vi "set_up_NS_queue.vi"(8 "error in (no error)":errorcluster, 10 "target":T1, 11 "StreamingBase in":refnum<class "StreamingBase.lvclass">) -> (0 "error out":errorcluster, 3 "StreamingBase out":refnum<class "StreamingBase.lvclass">)   [LabVIEW 2011, in "StreamingBase.lvclass"]
uses:
  StreamingBase.lvclass
  component_specification_cluster.ctl
  observer_cluster.ctl
  StreamingBase.lvclass/StreamingBase.ctl
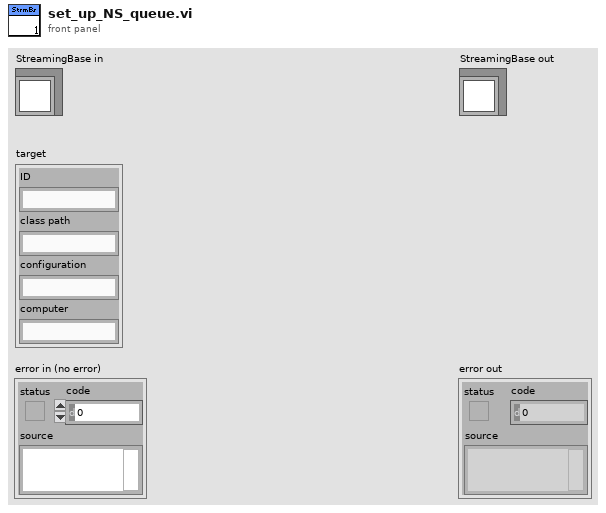
[diagram p1: front panel]
types:
  T1 = typedef "StreamingBase.lvclass/component_specification_cluster.ctl" = cluster{"ID":string, "class path":string, "configuration":string, "computer":string}
  T2 = typedef "StreamingBase.lvclass/observer_cluster.ctl" = cluster{"writer endpoint":refnum<k21>, "reader endpoint":refnum<k21>}
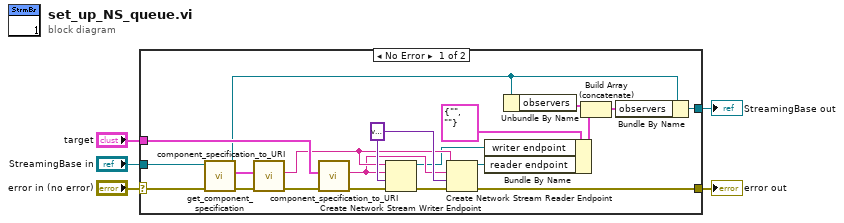
[diagram p0: block diagram]
diagram:
  n1 = case shown="No Error" "error in (no error)" {
    selector: "error in (no error)" -> [w25 w27]
    tunnel: [w22 w27] -> w4
    tunnel: [w6 w26] -> w2
    tunnel: "StreamingBase in" -> [w16 w26]
    tunnel: "target" -> [w17 _]
    frame No Error {
      w24 = variant ("variant")
      n2 = call-dynamic "get_component_specification.vi"("error in (no error)"=w25, "StreamingBase in"=w16) -> ("error out"=w21:errorcluster, "component specification"=w20:T1, "StreamingBase out"=w7:refnum<class "StreamingBase.lvclass">)  [unwired: 7 in]
      n3 = call "component_specification_to_URI.vi"("error in (no error)"=w21, "component specification"=w20) -> ("error out"=w19:errorcluster, "URI"=w15:string)  [unwired: 8 in]
      n4 = call "component_specification_to_URI.vi"("error in (no error)"=w19, "component specification"=w17) -> ("error out"=w18:errorcluster, "URI"=w14:string)  [unwired: 8 in]
      n5 = Create Network Stream Writer Endpoint(8:w18, 9:w24, 10:w14, 11:w15) -> (0:w23:errorcluster, 3:w11:refnum<k21>)  [unwired: 2 in]
      n6 = Create Network Stream Reader Endpoint(8:w23, 9:w24, 10:w14, 11:w15) -> (0:w22:errorcluster, 3:w10:refnum<k21>)  [unwired: 2 in]
      n7 = Bundle By Name(cluster=T2 {"writer endpoint"="", "reader endpoint"=""} ("observer"), "writer endpoint"=w11, "reader endpoint"=w10) -> (w9:T2)
      n8 = Unbundle By Name(w7) -> ("observers"=w13:T2[])
      n9 = Build Array (concatenate)(w13, w9) -> (w8:T2[])
      n10 = Bundle By Name(cluster=w7, "observers"=w8) -> (w6:refnum<class "StreamingBase.lvclass">)
    }
    frame Error {
    }
  }
  "error out" <- w4
  "StreamingBase out" <- w2
